vi "ToMatlabParam.vi"(8 "BaseName":string, 9 "IgnoreContainerName":bool, 11 "Value":variant) -> (3 "Matlab Param Data":T1[](array[typedef]))   [LabVIEW 2017]
uses:
  Types/MatlabDataBundle.ctl
  Types/MatlabDataType.ctl
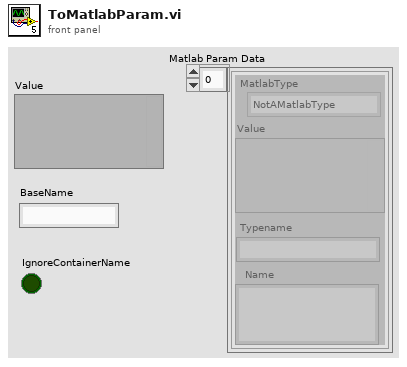
[diagram p1: front panel]
types:
  T1 = typedef "MatlabDataBundle.ctl" = cluster{"MatlabType":T2, "Value":variant, "Name":string, "Typename":string}
  T2 = typedef "MatlabDataType.ctl" = enum16{"NotAMatlabType", "Real", "Complex", "String", "Boolean"}
  T3 = typedef "NI_Data Type.lvlib/Data Type.ctl" = enum8{"Invalid Type", "Void", "I8", "I16", "I32", "I64", "U8", "U16", "U32", "U64", "Single Float", "Double Float", "Extended Float", "Single Complex", "Double Complex", "Extended Complex", "Enum U8", "Enum U16", "Enum U32", "Enum U64", "Single Float With Unit", "Double Float With Unit", "Extended Float With Unit", "Single Complex with Unit", "Double Complex with Unit", "Extended Complex with Unit", "Boolean", "String", "Path", "Picture", "Tag", "Array", "Cluster", "Variant", "LV Variant", "Waveform", "Timestamp", "Digital Waveform", "Digital Data", "ExpressData", "Refnum", "External Data", "VI", "Poly VI", "LabVIEW Class Instance", "Fixed Point"}
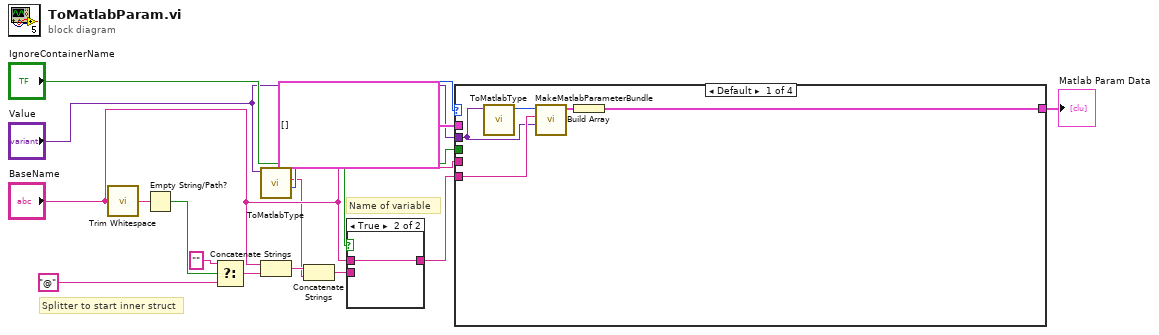
[diagram p0: block diagram]
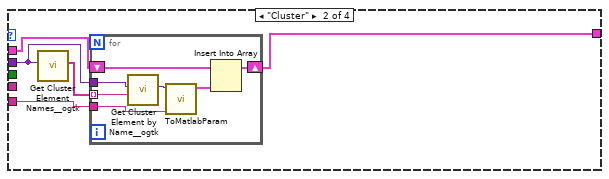
[diagram p3: hidden frame]
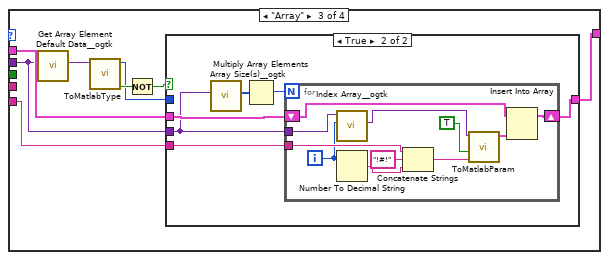
[diagram p4: hidden frame]
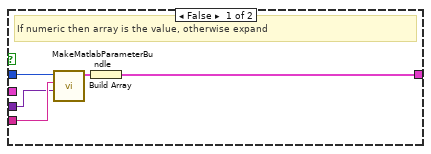
[diagram p5: hidden frame]
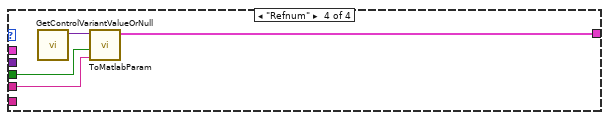
[diagram p6: hidden frame]
diagram:
  # "Splitter to start inner struct"
  # "Name of variable"
  n1 = call <vilib>:"Trim Whitespace.vi"("string"="BaseName") -> ("trimmed string"=w8:string)  [unwired: 1 in]
  n2 = Empty String/Path?(string/path=w8) -> (empty?=w7:bool)
  n3 = Select(t="" ("name"), s=w7, f="@" ("name")) -> (s? t:f=w15:string)
  n4 = call "ToMatlabType.vi"("Value"="Value") -> ("Type"=w2:T3, "Name"=w1:string)  [unwired: 7 in, 2 out]
  n5 = Concatenate Strings("BaseName", w15) -> (w9:string)
  n6 = Concatenate Strings(w9, w1) -> (w11:string)
  n7 = case shown="True" "IgnoreContainerName" {
    tunnel: [w16 w17] -> w12
    tunnel: w11 -> [w16 _]
    tunnel: "BaseName" -> [_ w17]
    frame False {
    }
    frame True {
    }
  }
  n8 = case shown="Default" w2 {
    tunnel: [w21 w27 w42 w65] -> w5
    tunnel: w12 -> [w19 w26 w39 _]
    tunnel: "IgnoreContainerName" -> [_ _ _ w66]
    tunnel: "BaseName" -> [_ _ _ w67]
    tunnel: T1[] [] -> [_ w24 w38 _]
    tunnel: "Value" -> [w18 w23 w36 _]
    frame Default {
      n9 = call "ToMatlabType.vi"("Value"=w18) -> ("MatlabType"=w20:T2)  [unwired: 7 in, 3 out]
      n10 = call "MakeMatlabParameterBundle.vi"("value"=w18, "name"=w19, "MatlabType"=w20) -> ("MatlabDataBundle"=w22:T1)  [unwired: 8 in]
      n11 = Build Array(w22) -> (w21:T1[])
    }
    frame "Cluster" {
      n12 = call <userlib>:"Get Cluster Element Names__ogtk.vi"("Cluster"=w23) -> ("Element Names"=w25:string[])  [unwired: 9 in, 1 out]
      n13 = for {
        shift-right: [w34] -> w27
        shift-left: w24 -> [w30]
        tunnel: w26 -> [w33]
        tunnel: w25 -> [w32] mode=indexing
        tunnel: w23 -> [w28]
        n14 = call <userlib>:"Get Cluster Element by Name__ogtk.vi"("Element Name"=w32, "Cluster"=w28) -> ("VElement"=w31:variant)  [unwired: 7 in, 2 out]
        n15 = call "ToMatlabParam.vi"("BaseName"=w33, "Value"=w31) -> ("Matlab Param Data"=w29:T1[])  [unwired: 9 in]
        n16 = Insert Into Array(array=w30, new element=w29) -> (w34:T1[])  [unwired: 1 in]
      }
    }
    frame "Array" {
      n17 = call <userlib>:"Get Array Element Default Data__ogtk.vi"("Array"=w36) -> ("Array Element Default Data"=w37:variant)  [unwired: 9 in, 1 out]
      n18 = call "ToMatlabType.vi"("Value"=w37) -> ("IsNumeric"=w41:bool, "MatlabType"=w35:T2)  [unwired: 7 in, 2 out]
      n19 = Not(x=w41) -> (.not. x?=w40:bool)
      n20 = case shown="True" w40 {
        tunnel: [w45 w53] -> w42
        tunnel: w39 -> [w47 w52]
        tunnel: w38 -> [_ w51]
        tunnel: w36 -> [w43 w48]
        tunnel: w35 -> [w44 _]
        frame False {
          # "If numeric then array is the value, otherwise expand"
          n21 = call "MakeMatlabParameterBundle.vi"("value"=w43, "name"=w47, "MatlabType"=w44) -> ("MatlabDataBundle"=w46:T1)  [unwired: 8 in]
          n22 = Build Array(w46) -> (w45:T1[])
        }
        frame True {
          n23 = call <userlib>:"Array Size(s)__ogtk.vi"("Array"=w48) -> ("Size(s)"=w50:u32[])  [unwired: 8 in, 2 out]
          n24 = Multiply Array Elements(1:w50) -> (0:w49:u32)
          n25 = for {
            N: w49 -> [_]
            shift-right: [w64] -> w53
            shift-left: w51 -> [w58]
            tunnel: w52 -> [w63]
            tunnel: w48 -> [w55]
            i -> [w56]
            n26 = call <userlib>:"Index Array__ogtk.vi"("Index (1D)"=w56, "MultiD Array"=w55) -> ("Array Element"=w54:variant)  [unwired: 8 in, 1 out]
            n27 = Number To Decimal String(number=w56) -> (decimal integer string=w61:string)  [unwired: 1 in]
            n28 = Concatenate Strings(w63, "!#!" ("string"), w61) -> (w60:string)
            n29 = call "ToMatlabParam.vi"("BaseName"=w60, "IgnoreContainerName"=TRUE, "Value"=w54) -> ("Matlab Param Data"=w57:T1[])  [unwired: 8 in]
            n30 = Insert Into Array(array=w58, new element=w57) -> (w64:T1[])  [unwired: 1 in]
          }
        }
      }
    }
    frame "Refnum" {
      n31 = call "GetControlVariantValueOrNull.vi"() -> ("Value"=w68:variant)  [unwired: 10 in, 1 out]
      n32 = call "ToMatlabParam.vi"("BaseName"=w67, "IgnoreContainerName"=w66, "Value"=w68) -> ("Matlab Param Data"=w65:T1[])  [unwired: 8 in]
    }
  }
  "Matlab Param Data" <- w5
